vi "Open System Definition.vi"(8 "error in (no error)":errorcluster, 11 "path":path) -> (0 "error out":errorcluster, 2 "System Node Paths":T1, 3 "SysDef Ref":T2)   [LabVIEW 2019, in "Simple SysDef API.lvlib"]
uses:
  <userlib>/SimpleSysDef/Simple SysDef API.lvlib
  <userlib>/SimpleSysDef/_SubVIs/System Definition Reference.ctl
  NationalInstruments.VeriStand.SystemDefinitionAPI
  <userlib>/SimpleSysDef/_SubVIs/System Node Paths.ctl
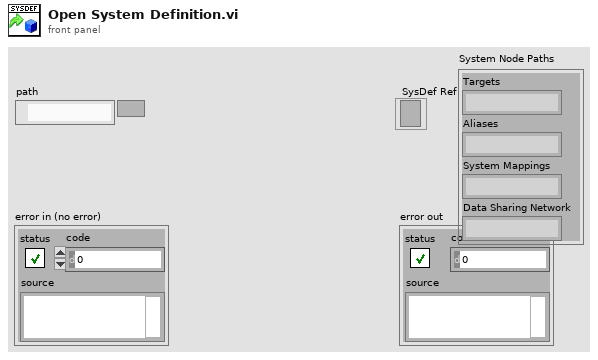
[diagram p1: front panel]
types:
  T1 = typedef "Simple SysDef API.lvlib/System Node Paths.ctl" = cluster{"Targets":string, "Aliases":string, "System Mappings":string, "Data Sharing Network":string}
  T2 = typedef "Simple SysDef API.lvlib/System Definition Reference.ctl" = refnum<k24>
  T3 = cluster{"[0]":string, "[1]":string, "[2]":string, "[3]":string}
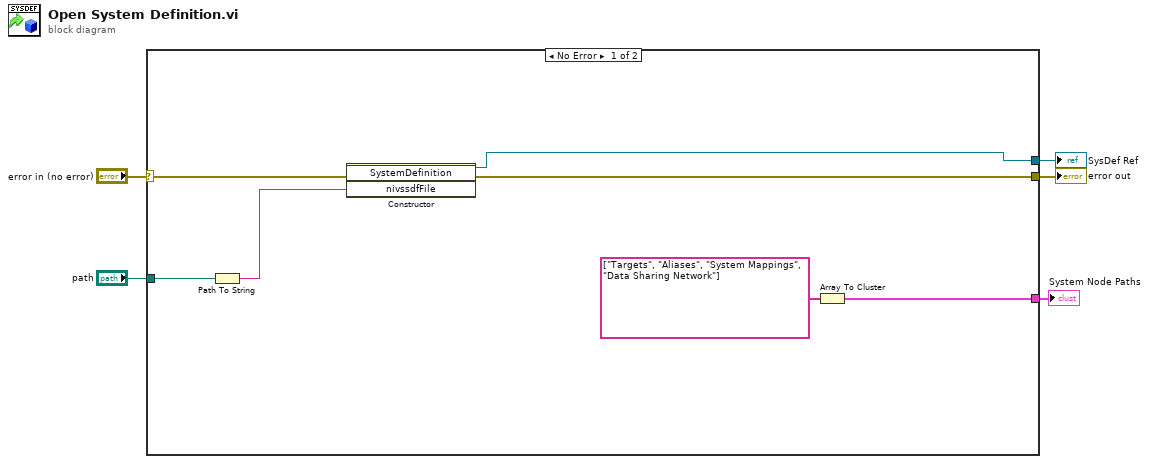
[diagram p0: block diagram]
diagram:
  n1 = case shown="No Error" "error in (no error)" {
    selector: "error in (no error)" -> [w6 w13]
    tunnel: "path" -> [w12 _]
    tunnel: [w7 w13] -> w4
    tunnel: [w8 _] -> w3
    tunnel: [w10 _] -> w1
    frame No Error {
      n2 = Path To String(path=w12) -> (string=w9:string)
      n3 = constructor class="SystemDefinition"(error in=w6, "nivssdfFile"=w9) -> (reference out=w8:refnum<k24>, error out=w7:errorcluster)  [unwired: 2 in, 2 out]
      n4 = Array To Cluster(array=string[] ["Targets", "Aliases", "System Mappings", "Data Sharing Network"]) -> (cluster=w10:T3)
    }
    frame Error {
    }
  }
  "error out" <- w4
  "SysDef Ref" <- w3
  "System Node Paths" <- w1
